vi "ex1c.vi"() -> ()   [LabVIEW 2022 SP3]
panel:
  out "output array":i32[][](array[numeric])
  in  "dimension size":i32
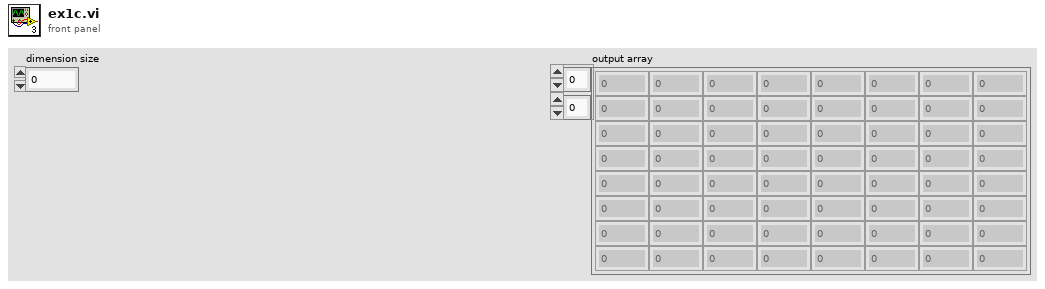
[diagram p1: front panel]
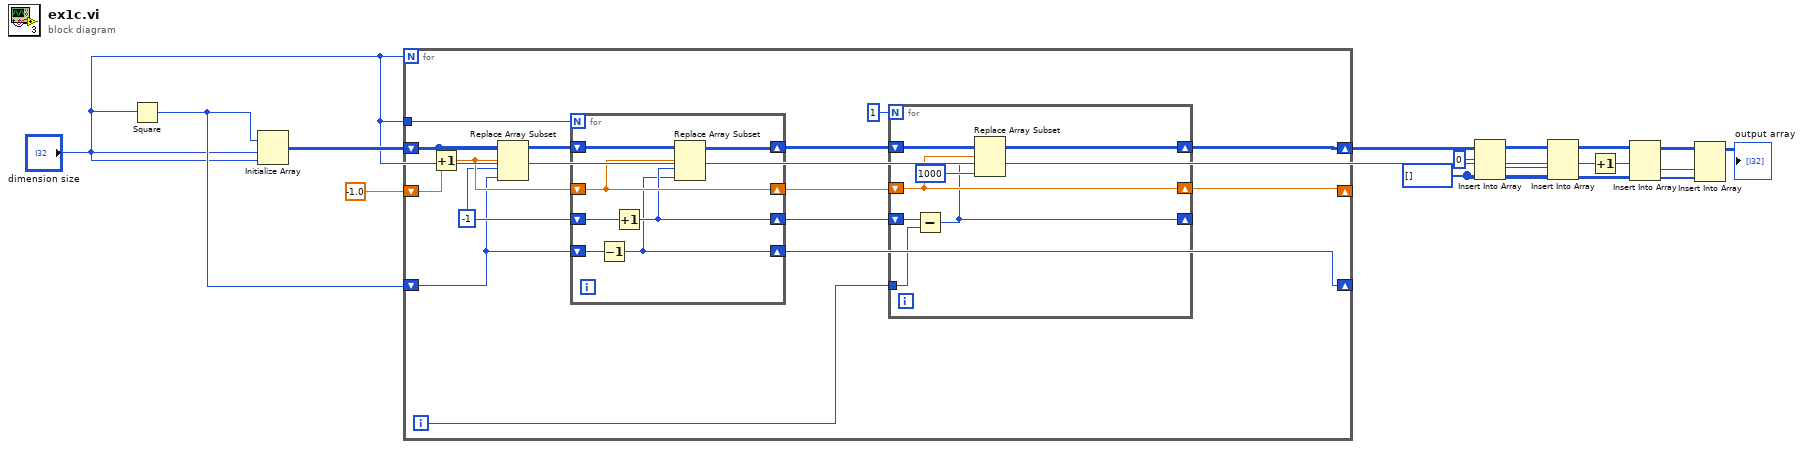
[diagram p0: block diagram]
diagram:
  w2 = i32[] [] ("new element/subarray")
  w7 = 0 ("index (row)")
  n1 = Square(x="dimension size") -> (x^2=w11:i32)
  n2 = Initialize Array(w11, "dimension size", "dimension size") -> (w12:i32[][])
  n3 = for {
    N: "dimension size" -> [_]
    shift-right: [w18] -> w9
    shift-left: w12 -> [w23]
    shift-right: [w16] -> _
    shift-left: w11 -> [w21]
    shift-right: [w17] -> _
    shift-left: -1.0 -> [w26]
    tunnel: "dimension size" -> [w22]
    i -> [w13]
    w24 = -1
    n4 = Increment(x=w26) -> (x+1=w25:dbl)
    n5 = Replace Array Subset(array=w23, new element=w21, index (row)=w25, index (col)=w24) -> ()  [unwired: 1 out]
    n6 = for {
      N: w22 -> [_]
      shift-right: [w36] -> w19
      shift-left: w25 -> [w36]
      shift-right: [w35] -> w14
      shift-left: w24 -> [w40]
      shift-right: [w37] -> w20
      shift-left: w23 -> [w39]
      shift-right: [w34] -> w16
      shift-left: w21 -> [w38]
      n7 = Decrement(x=w38) -> (x-1=w34:i32)
      n8 = Increment(x=w40) -> (x+1=w35:i32)
      n9 = Replace Array Subset(array=w39, new element=w34, index (row)=w36, index (col)=w35) -> (w37:i32[][])
    }
    n10 = for {
      N: 1 -> [_]
      shift-right: [w31] -> w18
      shift-left: w20 -> [w33]
      shift-right: [w30] -> w17
      shift-left: w19 -> [w30]
      shift-right: [w28] -> _
      shift-left: w14 -> [w27]
      tunnel: w13 -> [w29]
      n11 = Subtract(x=w27, y=w29) -> (x-y=w28:i32)
      n12 = Replace Array Subset(array=w33, new element=1000 ("new element/subarray"), index (row)=w30, index (col)=w28) -> (w31:i32[][])
    }
  }
  n13 = Insert Into Array(array=w9, index (row)=w7, new element=w2) -> (w8:i32[][])  [unwired: 1 in]
  n14 = Insert Into Array(array=w8, index (col)=w7, new element=w2) -> (w6:i32[][])  [unwired: 1 in]
  n15 = Increment(x="dimension size") -> (x+1=w3:i32)
  n16 = Insert Into Array(array=w6, index (row)=w3, new element=w2) -> (w4:i32[][])  [unwired: 1 in]
  n17 = Insert Into Array(array=w4, index (col)=w3, new element=w2) -> (→"output array":i32[][])  [unwired: 1 in]
